vi "Test Program milliGAT.vi"() -> ()   [LabVIEW 2018]
uses:
  VICI M6 M50 Party Mode.lvlib
  \\smbgbl.drmvfs102.pfizer.com\FAST_Team/Software/LabVIEW/Third Party Drivers/Third Party Drivers/VICI/Global FIA milliGAT.lvlib
  <vilib>/Platform/TimedLoop/XDataNode/XDataNode.xnode
  <vilib>/Platform/TimedLoop/XDataNode/nitl_modes.ctl
  <vilib>/Platform/TimedLoop/XDataNode/XDNodeRunTimeDep.lvlib
  <vilib>/Platform/TimedLoop/XDataNode/wakeup.ctl
  <vilib>/Platform/TimedLoop/XDataNode/timing_clust.ctl
  Settings Cluster.ctl
  \\smbgbl.drmvfs102.pfizer.com\FAST_Team/Software/LabVIEW/Third Party Drivers/Third Party Drivers/VICI/Public/Utility/Pump Address.ctl
panel:
  out "microliters/min":dbl
  out "Connection Error":bool
  out "error out":errorcluster
  in  "Pump ID (0:A)":T1
  in  "speed":dbl
  in  "VICI Settings":T2
  in  "stop":bool
  out "Pump On?":enum16{"Off", "On", "Not Initialized"}(ring)
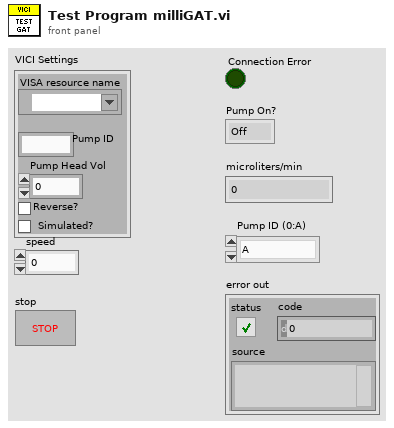
[diagram p1: front panel]
types:
  T1 = typedef "VICI M6 M50 Party Mode.lvlib/Global FIA milliGAT.lvlib/Pump Address.ctl" = enum16{"A", "B", "C", "D", "E", "F", "G", "H", "I", "J", "K", "L", "M", "N", "O", "P", "Q", "R", "S", "T", "U", "V", "W", "X", "Y", "Z", "a", "b", "c", "d", "e", "f", "g", "h", "i", "j", "k", "l", "m", "n", "o", "p", "q", "r", "s", "t", "u", "v", "w", "x", "y", "z", "0", "1", "2", "3", "4", "5", "6", "7", "8", "9"}
  T2 = typedef "VICI M6 M50 Party Mode.lvlib/Settings Cluster.ctl" = cluster{"VISA resource name":refnum<visa-resource-name>, "Pump ID":string, "Pump Head Vol":dbl, "Reverse?":bool, "Simulated?":bool}
  T3 = typedef "XDNodeRunTimeDep.lvlib/timing_clust.ctl" = cluster{"Expected End [f-1]":u64, "Actual End [f-1]":u64, "Finished Late? [f-1]":bool, "Expected End [i-1]":u64, "Actual End [i-1]":u64, "Finished Late? [i-1]":bool, "Expected Start [i]":u64, "Actual Start [i]":u64, "Expected Start [f]":u64, "Actual Start [f]":u64, "Source Name":string, "Structure Name":string, "Period":i64, "Deadline":i64, "Offset":i64, "Start":i64, "Priority":i32, "Timeout":i32, "Mode":T4, "Wakeup Reason":T5, "Error":errorcluster, "Source Type":string, "Secondary Source Type":string, "Global End Time":u64, "Global Start Time":u64, "Frame Duration":u64, "Iteration Duration":u64, "Assigned CPU":i32, "I/O Scan Engine Mode":u32}
  T4 = typedef "XDNodeRunTimeDep.lvlib/nitl_modes.ctl" = enum32{"No Change", "Process missed periods, maintain original phase", "Discard missed periods, maintain original phase", "Process missed periods, ignore original phase", "Discard missed periods, ignore original phase"}
  T5 = typedef "XDNodeRunTimeDep.lvlib/wakeup.ctl" = enum32{"Normal", "Aborted", "Asynchronous wakeup", "Timing source error", "Timed loop error", "Timeout"}
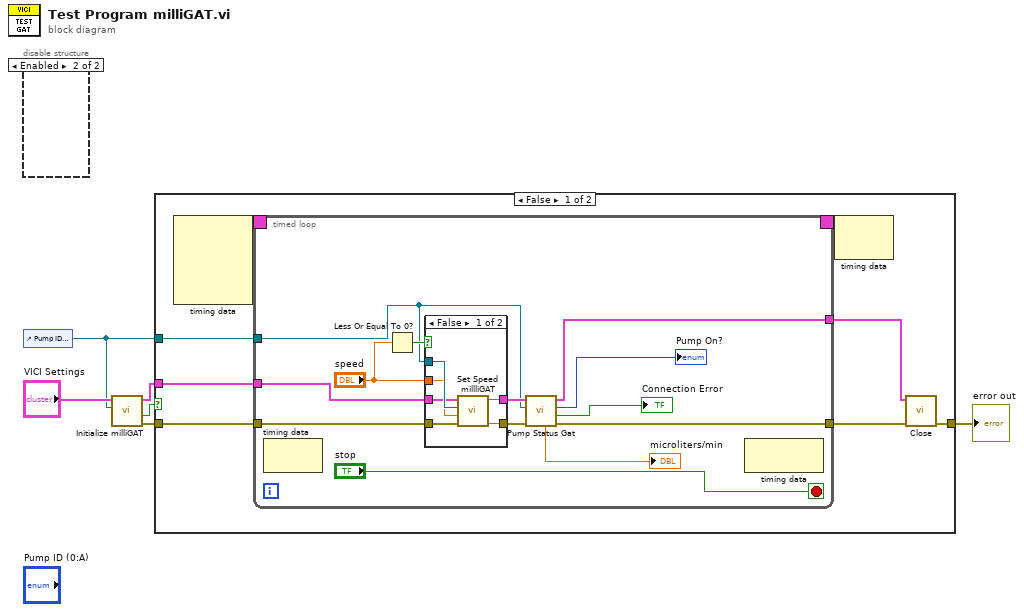
[diagram p0: block diagram]
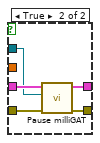
[diagram p2: hidden frame]
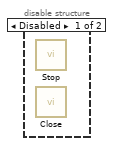
[diagram p4: hidden frame]
diagram:
  n1 = disable-structure shown="Enabled" {
    frame Disabled {
      n2 = call "Stop.vi"() -> ()  [unwired: 10 in, 2 out]
      n3 = call "Close.vi"() -> ()  [unwired: 11 in, 1 out]
    }
    frame Enabled {
    }
  }
  n4 = control-ref of="Pump ID (0:A)"() -> (w3:refnum<vi>)
  n5 = call "Initialize milliGAT.vi"("Enum in"=w3, "VICI Settings in"="VICI Settings") -> ("error out"=w5:errorcluster, "error?"=w1:bool, "VICI Settings out"=w6:T2)  [unwired: 7 in]
  n6 = case shown="False" w1 {
    tunnel: w6 -> [w12 _]
    tunnel: w5 -> [w11 w43]
    tunnel: w3 -> [w10 _]
    tunnel: [w9 w43] -> w2
    frame False {
      n7 = node-c288() -> (w8:T3)  [unwired: 4 in]
      n8 = timed-loop {
        tunnel: w12 -> [w23]
        tunnel: [w17] -> w14
        tunnel: w11 -> [w22]
        tunnel: [w27] -> w13
        tunnel: w10 -> [w18]
        timing: w8 -> [_]
        timing-out: [_] -> w7
        stop <- "stop" stop-if-true
        n9 = node-c288() -> ()  [unwired: 1 in, 1 out]
        n10 = Less Or Equal To 0?(x="speed") -> (x <= 0?=w26:bool)
        n11 = case shown="False" w26 {
          tunnel: w23 -> [w34 w40]
          tunnel: [w31 w37] -> w19
          tunnel: w22 -> [w32 w38]
          tunnel: [w30 w36] -> w24
          tunnel: "speed" -> [w33 _]
          tunnel: w18 -> [w35 w39]
          frame False {
            n12 = call "Set Speed millliGAT.vi"(8:w32, 9:w33, 10:w35, 11:w34) -> (0:w30, 3:w31)  [unwired: 6 in]
          }
          frame True {
            n13 = call "Pause milliGAT.vi"("error in (no error)"=w38, "Letter Enum"=w39, "VICI Settings in"=w40) -> ("error out"=w36:errorcluster, "VICI Settings out"=w37:T2)  [unwired: 7 in]
          }
        }
        n14 = call "Pump Status Gat.vi"("error in (no error)"=w24, "Enum in"=w18, "VICI Settings in"=w19) -> ("error out"=w27:errorcluster, "Connection Error"=→"Connection Error":bool, "Pump On?"=→"Pump On?":enum16{"Off", "On", "Not Initialized"}, "VICI Settings out"=w17:T2, "microliters/min"=→"microliters/min":dbl)  [unwired: 4 in]
        n15 = node-c288() -> ()  [unwired: 1 in, 1 out]
      }
      n16 = node-c288(w7) -> ()  [unwired: 1 out]
      n17 = call "Close.vi"("error in (no error)"=w13, "VICI Settings"=w14) -> ("error out"=w9:errorcluster)  [unwired: 7 in, 2 out]
    }
    frame True {
    }
  }
  "error out" <- w2
